vi "Carica immagine.vi"(5 "Immagine JPG":string) -> (0 "altezza":i16, 1 "larghezza":i16, 2 "Picture":picture)   [LabVIEW 2022 SP3]
uses:
  Labview/Globali.vi
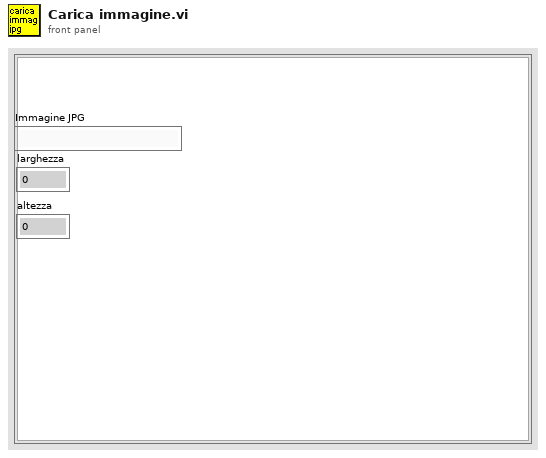
[diagram p1: front panel]
types:
  T1 = typedef "imagedata.ctl" = cluster{"image type":i32, "image depth":i32, "image":u8[], "mask":u8[], "colors":u32[], "Rectangle":cluster{"left":i16, "top":i16, "right":i16, "bottom":i16}}
  T2 = cluster{"left":i16, "top":i16, "right":i16, "bottom":i16}
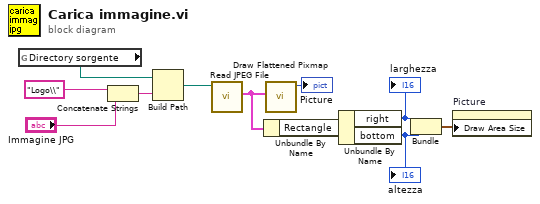
[diagram p0: block diagram]
diagram:
  n1 = global read "Globali.vi" "Directory sorgente"() -> (w7:path)
  n2 = Concatenate Strings("Logo\\", "Immagine JPG") -> (w8:string)
  n3 = Build Path(base path=w7, name or relative path=w8) -> (appended path=w11:path)
  n4 = call <vilib>:"Read JPEG File.vi"("path to JPEG file"=w11) -> ("image data"=w5:T1)  [unwired: 8 in, 2 out]
  n5 = Unbundle By Name(w5) -> ("Rectangle"=w6:T2)
  n6 = call <vilib>:"Draw Flattened Pixmap.vi"("image data"=w5) -> ("new picture"=→"Picture":picture)  [unwired: 8 in]
  n7 = Unbundle By Name(w6) -> ("right"=w3:i16, "bottom"=w2:i16)
  "altezza" <- w2
  "larghezza" <- w3
  n8 = Bundle("right"=w3, "bottom"=w2) -> (w4:cluster{"right":i16, "bottom":i16})  [unwired: 1 in]
  n9 = property on="Picture" class="Pict"("Draw Area Size"=w4) -> ()  [unwired: 2 in, 2 out]
